vi "Test MQTT-3.1.0-2.vi"(8 "error in (no error)":errorcluster) -> (0 "error out":errorcluster)   [LabVIEW 2013]
uses:
  source/Server/Connection/TCPConnection.lvclass
  source/Control Packets/ControlPacket/ControlPacket.lvclass
  <vilib>/addons/_JKI Toolkits/Caraya/classes/Test/Test.lvclass
  <vilib>/addons/_JKI Toolkits/Caraya/classes/Assert/Assert.lvclass
  source/Control Packets/CONNECT/CONNECT.lvclass
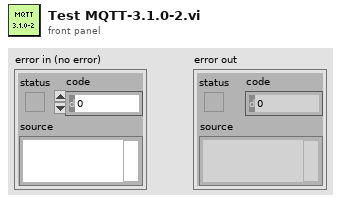
[diagram p1: front panel]
types:
  T1 = enum16{"Standard", "Buffered", "CRLF", "Immediate"}
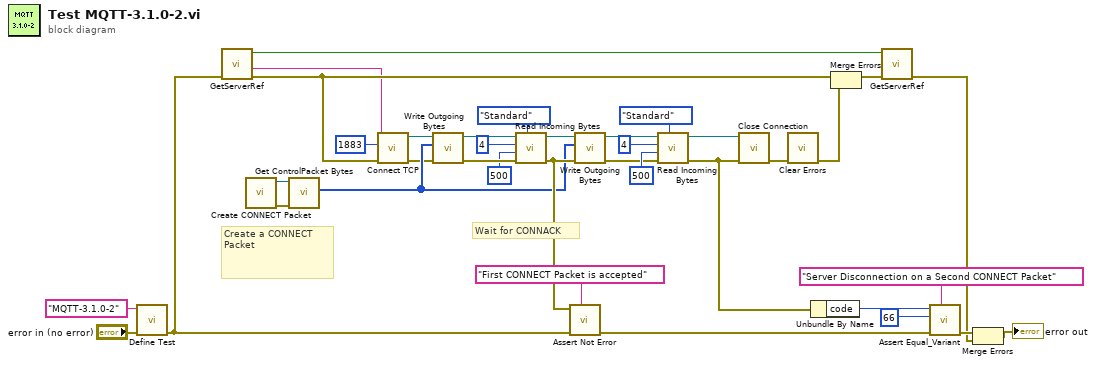
[diagram p0: block diagram]
diagram:
  # "Wait for CONNACK"
  # "Create a CONNECT Packet"
  n1 = call <vilib>:"Define Test.vi"("error in (no error)"="error in (no error)", "Label (VI Title)"="MQTT-3.1.0-2") -> ("error out"=w3:errorcluster)  [unwired: 9 in]
  n2 = call "GetServerRef.vi"("error in"=w3) -> ("error out"=w2:errorcluster, "Server address"=w1:string, "Created"=w6:bool)  [unwired: 7 in, 1 out]
  n3 = call "Create CONNECT Packet.vi"() -> ("error out"=w22:errorcluster, "CONNECT"=w23:refnum<class "CONNECT.lvclass">)  [unwired: 10 in]
  n4 = call "Get ControlPacket Bytes.vi"("error in (no error)"=w22, "ControlPacket"=w23) -> ("Bytes Stream"=w10:u8[])  [unwired: 7 in, 2 out]
  n5 = call "Connect TCP.vi"("error in (no error)"=w2, "remote port (80)"=u16 1883, "address (localhost)"=w1) -> ("error out"=w7:errorcluster, "TCPConnection out"=w8:refnum<class "TCPConnection.lvclass">)  [unwired: 7 in]
  n6 = call "Write Outgoing Bytes.vi"("error in (no error)"=w7, "Bytes"=w10, "TCPConnection in"=w8) -> ("error out"=w36:errorcluster, "TCPConnection out"=w37:refnum<class "TCPConnection.lvclass">)  [unwired: 7 in]
  n7 = call "Read Incoming Bytes.vi"("mode (standard)"=T1."Standard", "error in (no error)"=w36, "timeout (1000 ms)"=500 ("timeout ms (25000)"), "bytes to read (100)"=4 ("bytes to read"), "TCPConnection in"=w37) -> ("error out"=w13:errorcluster, "TCPConnection out"=w14:refnum<class "TCPConnection.lvclass">)  [unwired: 3 in, 2 out]
  n8 = call <vilib>:"Assert Not Error.vi"("Label"="First CONNECT Packet is accepted", "error in (no error)"=w3, "Not Error?"=w13) -> ("error out"=w21:errorcluster)  [unwired: 8 in]
  n9 = call "Write Outgoing Bytes.vi"("error in (no error)"=w13, "Bytes"=w10, "TCPConnection in"=w14) -> ("error out"=w16:errorcluster, "TCPConnection out"=w15:refnum<class "TCPConnection.lvclass">)  [unwired: 7 in]
  n10 = call "Read Incoming Bytes.vi"("mode (standard)"=T1."Standard", "error in (no error)"=w16, "timeout (1000 ms)"=500 ("timeout ms (25000)"), "bytes to read (100)"=4 ("bytes to read"), "TCPConnection in"=w15) -> ("error out"=w12:errorcluster, "TCPConnection out"=w11:refnum<class "TCPConnection.lvclass">)  [unwired: 3 in, 2 out]
  n11 = call-dynamic "Close Connection.vi"("error in (no error)"=w12, "TCPConnection in"=w11) -> ("error out"=w29:errorcluster)  [unwired: 8 in, 1 out]
  n12 = call <vilib>:"Clear Errors.vi"("error in (no error)"=w29) -> ("error out"=w24:errorcluster)  [unwired: 6 in]
  n13 = Unbundle By Name(w12) -> ("code"=w31:i32)
  n14 = Merge Errors(w2, w24) -> (w5:errorcluster)
  n15 = call "GetServerRef.vi"("error in"=w5, "Destroy (F)"=w6) -> ("error out"=w4:errorcluster)  [unwired: 6 in, 3 out]
  n16 = call <vilib>:"Assert Equal_Variant.vi"("Label"="Server Disconnection on a Second CONNECT Packet", "error in (no error)"=w21, "Y"=66 ("code"), "X"=w31) -> ("error out"=w34:errorcluster)  [unwired: 7 in]
  n17 = Merge Errors(w34, w4) -> (→"error out":errorcluster)
